vi "PH_Cam_BaseClass.check GUI object refs.vi"(0 "i ref in":refnum<vi>, 5 "error in (no error)":errorcluster) -> (14 "i ref out":refnum<vi>, 19 "error out":errorcluster)   [LabVIEW 2014]
doc: "This VI waits for the GUI indicator object refereces."
uses:
  PH_Cam_BaseClass.lvlib
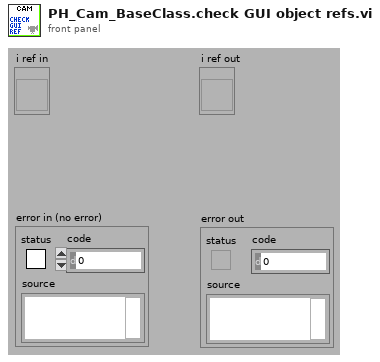
[diagram p1: front panel]
types:
  T1 = typedef "PH_Cam_BaseClass.lvlib/PH_Cam_BaseClass.i attribute.ctl" = cluster{"Gui Refs":T2, "Cam":cluster{"State":T3, "Source Notifier":refnum<notifier>, "Error":errorcluster, "Wanted Cam":string}, "Images":cluster{"Cam":T4, "Operation":T4, "PSDB":T4}, "Window Image":cluster{"Indicate Image":bool, "Window No.":i32, "Scale Facor":dbl, "Center Cross":bool, "Subtract Backgr":bool, "CoG":bool, "Color Palette":cluster{"Red":u8, "Green":u8, "Blue":u8}[], "Image On":bool}, "Default Prdc Int":i32, "Performance":cluster{"on":bool, "Timestamp Last Frame":i32}, "Histogram":cluster{"on":bool, "Mapping":bool}, "Save Image":cluster{"Save":bool, "File refnum":refnum<file>}, "Setting Service ID":i32, "Screen":cluster{"x-resolution":i16, "y-resolution":i16}, "On":bool, "Constructor finished":bool, "configured":bool}
  T2 = typedef "PH_Cam_BaseClass.lvlib/PH_Cam_BaseClass.GUI Refs.ctl" = cluster{"Frame Rate":refnum<vi>, "Get Frame Rate":refnum<vi>, "Camera State":refnum<vi>, "Show Image":refnum<vi>, "Get Histogram":refnum<vi>, "Mapping":refnum<vi>, "Histogram":refnum<vi>, "Center Cross":refnum<vi>, "Center of Gravity":refnum<vi>, "Scale Factor [%]":refnum<vi>, "Save Image":refnum<vi>, "Palette":refnum<vi>, "Camera State Bar":refnum<vi>, "Subtract Background":refnum<vi>, "Cam Error":refnum<vi>, "On":refnum<vi>, "Cam List":refnum<vi>}
  T3 = typedef "Device State.ctl" = i32
  T4 = typedef "IMAQ Image.ctl" = refnum<image>
  T5 = cluster{"Frame Rate":bool, "Get Frame Rate":bool, "Camera State":bool, "Show Image":bool, "Get Histogram":bool, "Mapping":bool, "Histogram":bool, "Center Cross":bool, "Center of Gravity":bool, "Scale Factor [%]":bool, "Save Image":bool, "Palette":bool, "Camera State Bar":bool, "Subtract Background":bool, "Cam Error":bool, "On":bool, "Cam List":bool}
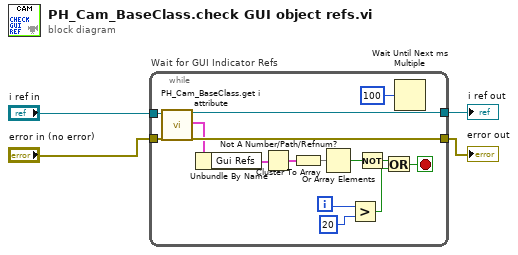
[diagram p0: block diagram]
diagram:
  n1 = while "Wait for GUI Indicator Refs" {
    tunnel: [w16] -> w4
    tunnel: "error in (no error)" -> [w14]
    tunnel: "i ref in" -> [w13]
    tunnel: [w12] -> w3
    i -> [w18]
    stop <- w11 stop-if-true
    n2 = call "PH_Cam_BaseClass.get i attribute.vi"("i ref in"=w13, "error in (no error)"=w14) -> ("i ref out"=w12:refnum<vi>, "i attribute"=w10:T1, "error out"=w16:errorcluster)  [unwired: 15 in]
    n3 = Unbundle By Name(w10) -> ("Gui Refs"=w6:T2)
    n4 = Not A Number/Path/Refnum?(number/path/refnum=w6) -> (NaN/Path/Refnum?=w7:T5)
    n5 = Cluster To Array(cluster=w7) -> (array=w5:bool[])
    n6 = Or Array Elements(Boolean array=w5) -> (logical OR=w9:bool)
    n7 = Greater?(x=w18, y=20) -> (0:w15:bool)
    n8 = Not(x=w9) -> (.not. x?=w8:bool)
    n9 = Or(x=w8, y=w15) -> (x .or. y?=w11:bool)
    n10 = Wait Until Next ms Multiple(millisecond multiple=u32 100) -> ()  [unwired: 1 out]
  }
  "error out" <- w4
  "i ref out" <- w3
